vi "SIAM_to_ScanControl.vi"(8 "error in (no error)":errorcluster, 11 "Script":T3(array[cluster])=[{"Delay 10µs"=50, "command"=4060086273, "P0"=3, "P1"=2, "P2"=0, "P3"=0, "P4"=0, "P5-ticket"=0}, {"Delay 10µs"=0, "command"=101711937, "P0"=0, "P1"=627200, "P2"=0, "P3"=0, "P4"=0, "P5-ticket"=0}, {"Delay 10µs"=0, "command"=102760513, "P0"=0, "P1"=3851400, "P2"=0, "P3"=0, "P4"=0, "P5-ticket"=0}, {"Delay 10µs"=0, "command"=3289190402, "P0"=0, "P1"=0, "P2"=0, "P3"=0, "P4"=0, "P5-ticket"=0}, {"Delay 10µs"=264, "command"=102760481, "P0"=0, "P1"=0, "P2"=-1047728, "P3"=0, "P4"=0, "P5-ticket"=0}, {"Delay 10µs"=0, "command"=4060086273, "P0"=2, "P1"=7, "P2"=0, "P3"=0, "P4"=0, "P5-ticket"=0}, {"Delay 10µs"=116, "command"=3489660929, "P0"=2097152, "P1"=2097152, "P2"=0, "P3"=0, "P4"=0, "P5-ticket"=0}, {"Delay 10µs"=0, "command"=3489660929, "P0"=1, "P1"=1, "P2"=0, "P3"=0, "P4"=0, "P5-ticket"=0}, {"Delay 10µs"=100, "command"=3489660929, "P0"=1, "P1"=0, "P2"=0, "P3"=0, "P4"=0, "P5-ticket"=0}, {"Delay 10µs"=12638, "command"=3289190402, "P0"=0, "P1"=0, "P2"=0, "P3"=0, "P4"=0, "P5-ticket"=0}, {"Delay 10µs"=0, "command"=102760465, "P0"=0, "P1"=0, "P2"=0, "P3"=12718148, "P4"=0, "P5-ticket"=0}, {"Delay 10µs"=0, "command"=101711889, "P0"=0, "P1"=0, "P2"=0, "P3"=679161, "P4"=0, "P5-ticket"=0}, {"Delay 10µs"=132, "command"=102760465, "P0"=0, "P1"=0, "P2"=0, "P3"=-12718148, "P4"=0, "P5-ticket"=0}, {"Delay 10µs"=0, "command"=101711889, "P0"=0, "P1"=0, "P2"=0, "P3"=-679161, "P4"=0, "P5-ticket"=0}, {"Delay 10µs"=132, "command"=102760465, "P0"=0, "P1"=0, "P2"=0, "P3"=0, "P4"=0, "P5-ticket"=0}, {"Delay 10µs"=0, "command"=101711889, "P0"=0, "P1"=0, "P2"=0, "P3"=0, "P4"=0, "P5-ticket"=0}, {"Delay 10µs"=12855, "command"=3489660929, "P0"=2097152, "P1"=0, "P2"=0, "P3"=0, "P4"=0, "P5-ticket"=0}, {"Delay 10µs"=70, "command"=4043379297, "P0"=-7, "P1"=2, "P2"=1, "P3"=0, "P4"=0, "P5-ticket"=514}, {"Delay 10µs"=50, "command"=104857729, "P0"=-25600, "P1"=0, "P2"=0, "P3"=0, "P4"=0, "P5-ticket"=0}, {"Delay 10µs"=0, "command"=4043379297, "P0"=-43, "P1"=3, "P2"=1, "P3"=0, "P4"=0, "P5-ticket"=515}, {"Delay 10µs"=50, "command"=104857729, "P0"=51200, "P1"=0, "P2"=0, "P3"=0, "P4"=0, "P5-ticket"=0}, {"Delay 10µs"=50, "command"=102760513, "P0"=0, "P1"=3840000, "P2"=0, "P3"=0, "P4"=0, "P5-ticket"=0}, {"Delay 10µs"=10, "command"=4027518991, "P0"=0, "P1"=0, "P2"=0, "P3"=0, "P4"=0, "P5-ticket"=112}] {"command" format="%x" items=["read_x-Motor_status_ticket"=17305600, "init_x-Motor"=17760263, "read_x-Motor_absolute_ticket"=16781312, "move_x-Motor_absolute"=16777217, "move_x-Motor_relative"=16842753, "read_x-Motor_speed"=16977920, "set_x-Motor_speed"=16973825, "read_y-Motor_status_ticket"=18354176, "init_y-Motor"=18808839, "read_y-Motor_absolute_ticket"=17829888, "move_y-Motor_absolute"=17825793, "move_y-Motor_relative"=17891329, "read_y-Motor_speed"=18026496, "set_y-Motor_speed"=18022401, "read_z-Motor_status_ticket"=19402752, "init_z-Motor"=19857415, "stop_z-Motor"=19857423, "start_z-Motor"=19857422, "read_z-Motor_absolute_ticket"=18878464, "move_z-Motor_absolute"=18874369, "move_z-Motor_relative"=18939905, "read_Objective_status_ticket"=20451328, "init_Objective"=20905991, "read_Objective_absolute_ticket"=19927040, "move_Objective_absolute"=19922945, "move_Objective_relative"=19988481, "read_Objective-Motor_speed"=20123648, "set_Objective-Motor_speed"=20119553, "read_Filter_status_ticket"=21499904, "init_Filter"=21954567, "read_Filter_absolute_ticket"=20975616, "move_Filter_absolute"=20971521, "move_Filter_relative"=21037057, "read_Filter-Motor_speed"=21172224, "set_Filter-Motor_speed"=21168129, "read_Trans-Rad_status_ticket"=22548480, "init_Trans-Rad"=23003143, "read_Trans-Rad_absolute_ticket"=22024192, "move_Trans-Rad_absolute"=22020097, "move_Trans-Rad_relative"=22085633, "read_Trans-Motor_speed"=22220800, "set_Trans-Motor_speed"=22216705, "read_FRET_status_ticket"=23597056, "init_FRET"=24051719, "read_FRET_absolute_ticket"=23072768, "move_FRET_absolute"=23068673, "move_FRET_relative"=23134209, "read_FRET-Motor_speed"=23269376, "set_FRET-Motor_speed"=23265281, "read_SI-Rad_status_ticket"=24645632, "init_SI-Rad"=25100295, "read_SI-Rad_absolute_ticket"=24121344, "move_SI-Rad_absolute"=24117249, "move_SI-Rad_relative"=24182785, "read_SI-Rad_speed"=24317952, "set_SI-Rad_speed"=24313857, "I2C-write"=335544337, "I2C-read"=335548433, "UART0-VC-Baud-write"=469958673, "UART0-VC-Baud-read"=469962768, "UART0-VC-write"=469762065, "UART0-VC-write-Var"=469762067, "UART0-VC-read"=469766160, "UART0-VC-read-Var"=469766162, "UART1-TSM-Baud-read"=486739984, "UART1-TSM-write"=486539281, "UART1-TSM-write-ticket"=486543377, "UART1-TSM-write-var-binary"=486539283, "UART1-TSM-write-var-binary-ticket"=486543379, "UART1-TSM-read"=486543376, "UART1-TSM-read-var-binary"=486543378, "UART2-write"=503316497, "UART2-read"=503320592, "USB-UART0-write"=536870929, "USB-UART0-read"=536875024, "USB-UART0-Float-Bitschift"=537133073, "USB-UART0-read-Float"=536875234, "USB-UART0-write-Float"=536871139, "USB-UART0-read-Float"=536875250, "USB-UART0-write-Float"=536871155, "end_no_ticket"=4027514895, "end_ticket"=4027518991, "NoOp"=4060086272, "IO-read_bank0"=3489665024, "IO-write_bank0"=3489660929, "IO-read_bank1"=3506442240, "IO-write_bank1"=3506438145, "DA0-0_LED365"=2684354561, "DA0-1_LED385"=2685403137, "DA0-2_LED440"=2686451713, "DA0-3_LED470"=2687500289, "DA0-4_LED510"=2688548865, "DA0-5_LED550"=2689597441, "DA0-6_LED590"=2690646017, "DA0-7_LED640"=2691694593, "DA1-0_LED-R"=2701131777, "DA1-1_LED-G"=2702180353, "DA1-2_LED-B"=2703228929, "DA1-3_LED-AF"=2704277505, "DA1-4"=2705326081, "DA1-5"=2706374657, "DA1-6"=2707423233, "DA1-7"=2708471809, "DA2-Laser0"=2717908993, "DA2-Laser1"=2718957569, "DA2-Laser2"=2720006145, "DA2-Laser3"=2721054721, "DA2-Laser4"=2722103297, "Analog-read_AD0-0"=2818576384, "Analog-read-store_AD0-0"=2818572290, "IO-delay_bank0"=3489923073, "IO-delay_bank0_fromVar"=3489923075, "read_cam_clock"=3289124864, "store_cam_clock"=3289120770, "read_cam_phase"=3289190400, "store_cam_phase"=3289186306, "store_cam_phase-t"=3289190402, "Read ticks"=4026535936, "Read ticks to var"=4026535938, "Read IP"=4043313152, "Read IP into var"=4043313154, "Set IP from var"=4043309059, "Set IP from var, relative"=4043313155, "branchRel_if_equal"=4043374849, "decrement_branchRel_if_equal"=4043374945, "decrement_branchRel_if_greaterequal"=4043375201, "decrement_branchRel_if_greaterequal_withTicket"=4043379297, "decrement_branchRel_if_smaller"=4043375457, "increment_branchRel_if_smaller"=4043375473, "readVar"=4060090368, "writeVar"=4060086273, "copyVar0_from_var1"=4060086275, "math_addToVariable"=4076863488, "math_addVToVariable"=4076863489, "math_subToVariable"=4076863490, "math_subVToVariable"=4076863491, "math_multToVariable"=4076863492, "math_multvToVariable"=4076863493, "math_divideToVariable"=4076863494, "math_divideVToVariable"=4076863495, "math_modToVariable"=4076863496, "math_modVToVariable"=4076863497, "logic_and"=4093640704, "logic_or"=4093640706, "logic_xor"=4093640708, "bitshift"=4093640712, "set_1Galvo"=101712113, "set_x-Galvo"=102760689, "set_y-Galvo"=103809265, "set_z-Fokus"=104857841, "set_1Galvo_position-only"=101711937, "set_x-Galvo_position-only"=102760513, "set_y-Galvo_position-only"=103809089, "set_z-Fokus_position-only"=104857665, "set_x-Galvo_position-only_ticket"=102764609, "set_y-Galvo_position-only_ticket"=103813185, "set_z-Fokus_position-only_ticket"=104861761, "set_1Galvo_relativ-only"=101712001, "set_x-Galvo_relativ-only"=102760577, "set_y-Galvo_relativ-only"=103809153, "set_z-Fokus_relativ-only"=104857729, "set_1Galvo_speed-only"=101711905, "set_x-Galvo_speed-only"=102760481, "set_y-Galvo_speed-only"=103809057, "set_z-Fokus_speed-only"=104857633, "set_1Galvo_acc-only"=101711889, "set_x-Galvo_acc-only"=102760465, "set_y-Galvo_acc-only"=103809041, "set_z-Fokus_acc-only"=104857617, "read_1Galvo_ticket"=101716032, "read_x-Galvo_ticket"=102764608, "read_y-Galvo_ticket"=103813184, "read_z-Focus_ticket"=104861760, "x-Galvo_pos_fromVar"=102760515, "y-Galvo_pos_fromVar"=103809091, "z-Focus_pos_fromVar"=104857667, "Servo0"=67108865, "Servo0-enable"=68091911, "Servo0-disable"=68091919, "Servo1"=68157441, "Servo1-enable"=69140487, "Servo1-disable"=69140495, "Servo2-enable"=70189063, "Servo2"=69206017, "Servo3-enable"=71237639, "Servo3"=70254593, "x-ssi-init"=202309639, "x-ssi-disable"=202309647, "x-ssi-Bits"=201523201, "x-ssi-Read"=201330688, "x-ssi-ReadToVar"=201326594, "x-ssi-ReadToVar-ticket"=201330690, "y-ssi-init"=203358215, "y-ssi-disable"=203358223, "y-ssi-Bits"=202571777, "y-ssi-Read"=202379264, "y-ssi-ReadToVar"=202375170, "y-ssi-ReadToVat-ticket"=202379266]}) -> (0 "error out":errorcluster, 2 "Total 10µs ticks":u32=1000000, 3 "ScanSteuerung":T6(array[cluster])=[{"Time [10µs]"=0.0, "action"=enum."Abs", "channel"=enum."Digital", "value (/s)"=7.0}, {"Time [10µs]"=0.0, "action"=enum."LoopStart", "channel"=enum."Loop", "value (/s)"=10.0}, {"Time [10µs]"=50000.0, "action"=enum."Abs", "channel"=enum."Digital", "value (/s)"=1.0}, {"Time [10µs]"=100000.0, "action"=enum."Rel", "channel"=enum."GalvoX", "value (/s)"=2.0}, {"Time [10µs]"=100000.0, "action"=enum."LoopEnd", "channel"=enum."Loop", "value (/s)"=0.0}])   [LabVIEW 2011]
uses:
  ScanControl_Action.ctl
  ScanControl_Channel.ctl
  Drivers/SIAM/SIAM_command.ctl
panel:
  out "loopstarts":T1(array[cluster])
  in  "Hack, valid loopvars":u16[](array[numeric])=[2, 3]
  out "Last Command":i32
  # "OK working\ntodo \nloop var detect\ncorrect loop times  from jump points"
  # "relative timing"
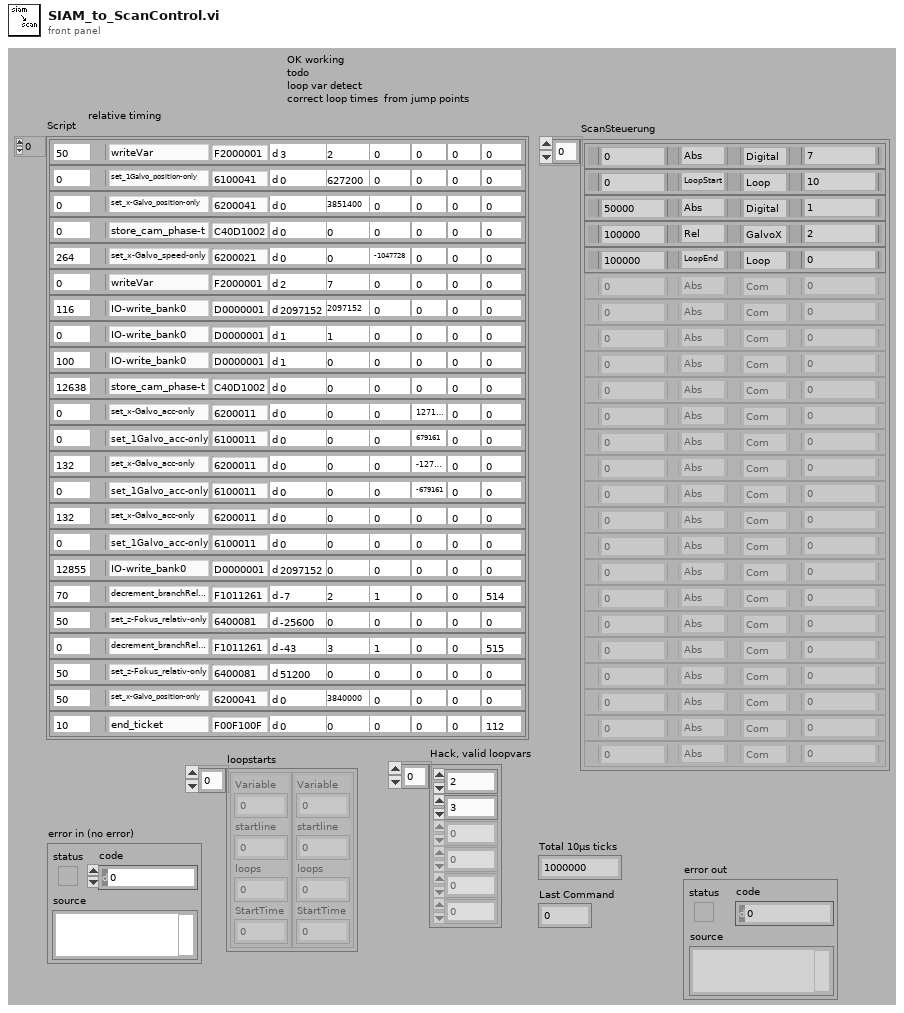
[diagram p1: front panel]
types:
  T1 = cluster{"Variable":i32, "startline":i32, "loops":i32, "StartTime":u64}[]
  T2 = typedef "SIAM_command.ctl" = u32
  T3 = cluster{"Delay 10µs":u32, "command":T2, "P0":i32, "P1":i32, "P2":i32, "P3":i32, "P4":i32, "P5-ticket":i32}[]
  T4 = typedef "ScanControl_Action.ctl" = enum16{"Abs", "Rel", "Inc", "IncInc", "LoopStart", "LoopEnd", "WaitTriggerRising"}
  T5 = typedef "ScanControl_Channel.ctl" = enum16{"Com", "AnalogConfig", "AnalogValue", "GalvoX", "GalvoY", "Galvo3", "Galvo4", "Digital", "Free", "Loop", "SMoveTime", "Image1X", "Image1Y", "Image2X", "Image2Y"}
  T6 = cluster{"Time [10µs]":dbl, "action":T4, "channel":T5, "value (/s)":dbl}[]
  T7 = cluster{"Time [10µs]":dbl, "action":T4, "channel":T5, "value (/s)":dbl}
  T8 = cluster{"Variable":i32, "startline":i32, "loops":i32, "StartTime":i32}[]
  T9 = enum16{"Com", "AnalogConfig", "AnalogValue", "GalvoX", "GalvoY", "Galvo3", "Galvo4", "Digital", "Free", "Loop", "SMoveTime", "Image1X", "Image1Y", "Image2X", "Image2Y"}[]
  T10 = enum8{"Ch0", "Ch1", "x-Galvo", "y-Galvo", "z-Focus"}
  T11 = cluster{"P0":i32, "startline":i32, "P1":i32, "StartTime":u64}[]
  T12 = cluster{"Variable":i32, "startline":i32, "loops":i32, "StartTime":u64}
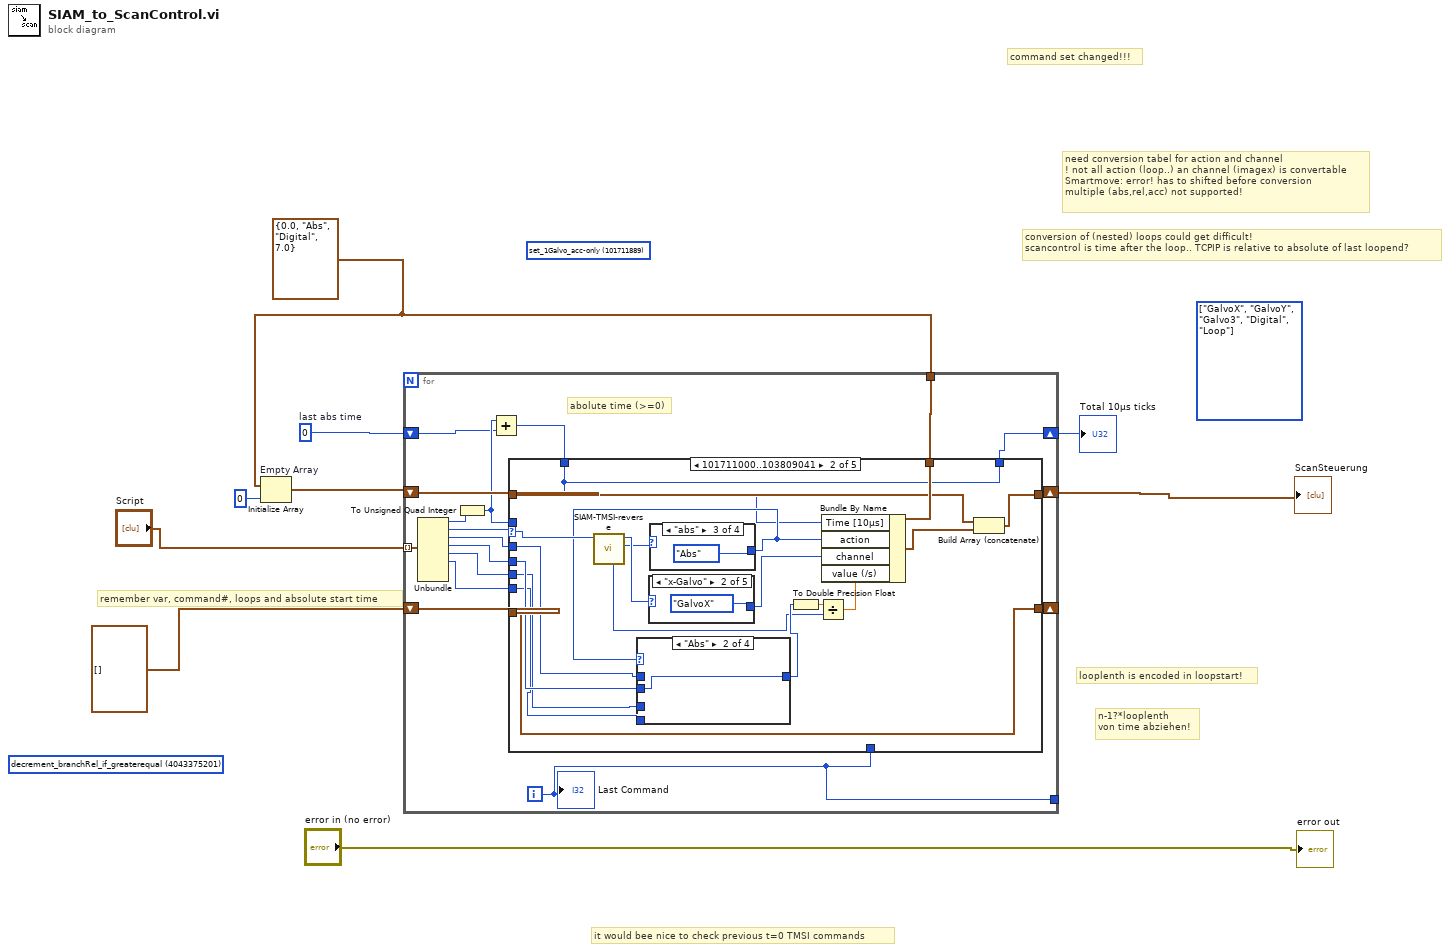
[diagram p0: block diagram]
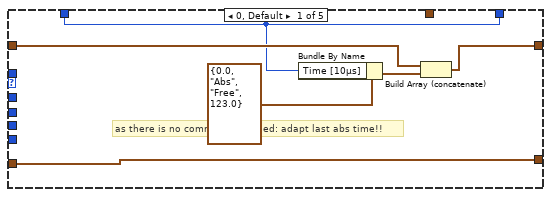
[diagram p2: hidden frame]
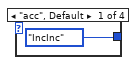
[diagram p6: hidden frame]
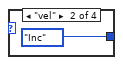
[diagram p7: hidden frame]
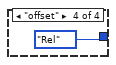
[diagram p8: hidden frame]
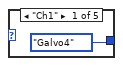
[diagram p9: hidden frame]
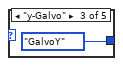
[diagram p10: hidden frame]
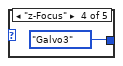
[diagram p11: hidden frame]
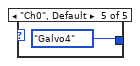
[diagram p12: hidden frame]
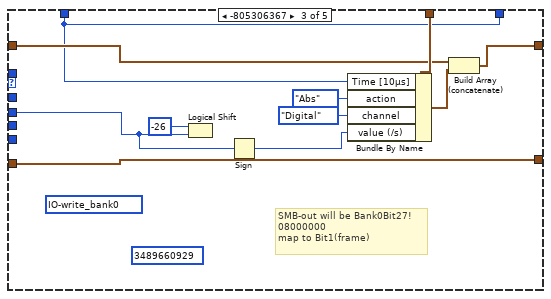
[diagram p13: hidden frame]
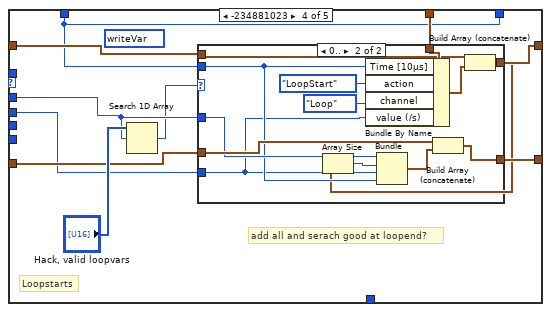
[diagram p14: hidden frame]
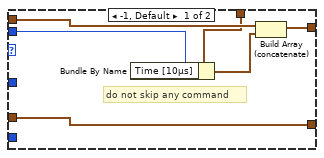
[diagram p15: hidden frame]
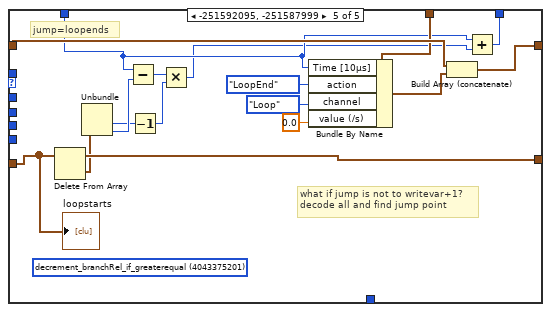
[diagram p16: hidden frame]
diagram:
  (unwired) T2 4043375201 items=["read_x-Motor_status_ticket"=17305600, "init_x-Motor"=17760263, "read_x-Motor_absolute_ticket"=16781312, "move_x-Motor_absolute"=16777217, "move_x-Motor_relative"=16842753, "read_y-Motor_status_ticket"=18354176, "init_y-Motor"=18808839, "read_y-Motor_absolute_ticket"=17829888, "move_y-Motor_absolute"=17825793, "move_y-Motor_relative"=17891329, "read_z-Motor_status_ticket"=19402752, "init_z-Motor"=19857415, "stop_z-Motor"=19857423, "start_z-Motor"=19857422, "read_z-Motor_absolute_ticket"=18878464, "move_z-Motor_absolute"=18874369, "move_z-Motor_relative"=18939905, "end_no_ticket"=4027514895, "end_ticket"=4027518991, "IO-read_bank0"=218107904, "IO-write_bank0"=218103809, "IO-read_bank1"=219156480, "IO-write_bank1"=219152385, "IO-delay_bank0"=218365953, "IO-delay_bank0_fromVar"=218365955, "read_cam_clock"=3289124864, "store_cam_clock"=3289120770, "read_cam_phase"=3289190400, "set_cam_deadtime"=3288989697, "set_cam_10uscycles"=3289055233, "set_cam_10uscycles_fromVariable"=3289055235, "calc_cam"=3289317386, "store_cam_Var"=3289251842, "math_addToVariable"=4060086278, "readVar"=4060090368, "writeVar"=4060086273, "copyVar"=4060086276, "decrement_branchRel_if_equal"=4043374945, "decrement_branchRel_if_greaterequal"=4043375201, "decrement_branchRel_if_greaterequal_withTicket"=4043379297, "decrement_branchRel_if_smaller"=4043375457, "increment_branchRel_if_smaller"=4043375473, "writeTMSI"=100663297, "writeTMSI_fromVar"=100663299] ("command")
  (unwired) T2 101711889 items=["read_x-Motor_status_ticket"=17305600, "init_x-Motor"=17760263, "read_x-Motor_absolute_ticket"=16781312, "move_x-Motor_absolute"=16777217, "move_x-Motor_relative"=16842753, "read_x-Motor_speed"=16977920, "set_x-Motor_speed"=16973825, "read_y-Motor_status_ticket"=18354176, "init_y-Motor"=18808839, "read_y-Motor_absolute_ticket"=17829888, "move_y-Motor_absolute"=17825793, "move_y-Motor_relative"=17891329, "read_y-Motor_speed"=18026496, "set_y-Motor_speed"=18022401, "read_z-Motor_status_ticket"=19402752, "init_z-Motor"=19857415, "stop_z-Motor"=19857423, "start_z-Motor"=19857422, "read_z-Motor_absolute_ticket"=18878464, "move_z-Motor_absolute"=18874369, "move_z-Motor_relative"=18939905, "read_Objective_status_ticket"=20451328, "init_Objective"=20905991, "read_Objective_absolute_ticket"=19927040, "move_Objective_absolute"=19922945, "move_Objective_relative"=19988481, "read_Objective-Motor_speed"=20123648, "set_Objective-Motor_speed"=20119553, "read_Filter_status_ticket"=21499904, "init_Filter"=21954567, "read_Filter_absolute_ticket"=20975616, "move_Filter_absolute"=20971521, "move_Filter_relative"=21037057, "read_Filter-Motor_speed"=21172224, "set_Filter-Motor_speed"=21168129, "read_Trans-Rad_status_ticket"=22548480, "init_Trans-Rad"=23003143, "read_Trans-Rad_absolute_ticket"=22024192, "move_Trans-Rad_absolute"=22020097, "move_Trans-Rad_relative"=22085633, "read_Trans-Motor_speed"=22220800, "set_Trans-Motor_speed"=22216705, "read_FRET_status_ticket"=23597056, "init_FRET"=24051719, "read_FRET_absolute_ticket"=23072768, "move_FRET_absolute"=23068673, "move_FRET_relative"=23134209, "read_FRET-Motor_speed"=23269376, "set_FRET-Motor_speed"=23265281, "read_SI-Rad_status_ticket"=24645632, "init_SI-Rad"=25100295, "read_SI-Rad_absolute_ticket"=24121344, "move_SI-Rad_absolute"=24117249, "move_SI-Rad_relative"=24182785, "read_SI-Rad_speed"=24317952, "set_SI-Rad_speed"=24313857, "I2C-write"=335544337, "I2C-read"=335548433, "UART0-VC-Baud-write"=469958673, "UART0-VC-Baud-read"=469962768, "UART0-VC-write"=469762065, "UART0-VC-write-Var"=469762067, "UART0-VC-read"=469766160, "UART0-VC-read-Var"=469766162, "UART1-TSM-Baud-read"=486739984, "UART1-TSM-write"=486539281, "UART1-TSM-write-ticket"=486543377, "UART1-TSM-write-var-binary"=486539283, "UART1-TSM-write-var-binary-ticket"=486543379, "UART1-TSM-read"=486543376, "UART1-TSM-read-var-binary"=486543378, "UART2-write"=503316497, "UART2-read"=503320592, "USB-UART0-write"=536870929, "USB-UART0-read"=536875024, "USB-UART0-Float-Bitschift"=537133073, "USB-UART0-read-Float"=536875234, "USB-UART0-write-Float"=536871139, "USB-UART0-read-Float"=536875250, "USB-UART0-write-Float"=536871155, "end_no_ticket"=4027514895, "end_ticket"=4027518991, "IO-read_bank0"=3489665024, "IO-write_bank0"=3489660929, "IO-read_bank1"=3506442240, "IO-write_bank1"=3506438145, "DA0-0_LED365"=2684354561, "DA0-1_LED385"=2685403137, "DA0-2_LED440"=2686451713, "DA0-3_LED470"=2687500289, "DA0-4_LED510"=2688548865, "DA0-5_LED550"=2689597441, "DA0-6_LED590"=2690646017, "DA0-7_LED640"=2691694593, "DA1-0_LED-R"=2701131777, "DA1-1_LED-G"=2702180353, "DA1-2_LED-B"=2703228929, "DA1-3_LED-AF"=2704277505, "DA1-4"=2705326081, "DA1-5"=2706374657, "DA1-6"=2707423233, "DA1-7"=2708471809, "DA2-Laser0"=2717908993, "DA2-Laser1"=2718957569, "DA2-Laser2"=2720006145, "DA2-Laser3"=2721054721, "DA2-Laser4"=2722103297, "Analog-read_AD0-0"=2818576384, "Analog-read-store_AD0-0"=2818572290, "IO-delay_bank0"=3489923073, "IO-delay_bank0_fromVar"=3489923075, "read_cam_clock"=3289124864, "store_cam_clock"=3289120770, "read_cam_phase"=3289190400, "store_cam_phase"=3289186306, "store_cam_phase-t"=3289190402, "Read ticks"=4027518976, "Read ticks to var"=4027518978, "Read IP"=4043313152, "Read IP into var"=4043313154, "Set IP from var"=4043309059, "Set IP from var, relative"=4043313155, "decrement_branchRel_if_equal"=4043374945, "decrement_branchRel_if_greaterequal"=4043375201, "decrement_branchRel_if_greaterequal_withTicket"=4043379297, "decrement_branchRel_if_smaller"=4043375457, "increment_branchRel_if_smaller"=4043375473, "readVar"=4060090368, "writeVar"=4060086273, "copyVar0_from_var1"=4060086275, "math_addToVariable"=4076863488, "math_addVToVariable"=4076863489, "math_subToVariable"=4076863490, "math_subVToVariable"=4076863491, "math_multToVariable"=4076863492, "math_multvToVariable"=4076863493, "math_divideToVariable"=4076863494, "math_divideVToVariable"=4076863495, "math_modToVariable"=4076863496, "math_modVToVariable"=4076863497, "logic_and"=4093640704, "logic_or"=4093640706, "logic_xor"=4093640708, "bitshift"=4093640712, "set_1Galvo"=101712113, "set_x-Galvo"=102760689, "set_y-Galvo"=103809265, "set_z-Fokus"=104857841, "set_1Galvo_position-only"=101711937, "set_x-Galvo_position-only"=102760513, "set_y-Galvo_position-only"=103809089, "set_z-Fokus_position-only"=104857665, "set_x-Galvo_position-only_ticket"=102764609, "set_y-Galvo_position-only_ticket"=103813185, "set_z-Fokus_position-only_ticket"=104861761, "set_1Galvo_relativ-only"=101712001, "set_x-Galvo_relativ-only"=102760577, "set_y-Galvo_relativ-only"=103809153, "set_z-Fokus_relativ-only"=104857729, "set_1Galvo_speed-only"=101711905, "set_x-Galvo_speed-only"=102760481, "set_y-Galvo_speed-only"=103809057, "set_z-Fokus_speed-only"=104857633, "set_1Galvo_acc-only"=101711889, "set_x-Galvo_acc-only"=102760465, "set_y-Galvo_acc-only"=103809041, "set_z-Fokus_acc-only"=104857617, "read_1Galvo_ticket"=101716032, "read_x-Galvo_ticket"=102764608, "read_y-Galvo_ticket"=103813184, "read_z-Focus_ticket"=104861760, "x-Galvo_pos_fromVar"=102760515, "y-Galvo_pos_fromVar"=103809091, "z-Focus_pos_fromVar"=104857667, "Servo0"=67108865, "Servo0-enable"=68091911, "Servo0-disable"=68091919, "Servo1"=68157441, "Servo1-enable"=69140487, "Servo1-disable"=69140495, "Servo2-enable"=70189063, "Servo2"=69206017, "Servo3-enable"=71237639, "Servo3"=70254593, "xEncoder-Enable"=202309639, "xEncoder-Bits"=201523201, "xEncoder-Read"=201330688, "xEncoder-Read"=201326594, "xEncoder-Read-ticket"=201330690, "yEncoder-Enable"=203358215, "yEncoder-Bits"=202571777, "yEncoder-Read"=202379264, "yEncoder-Read"=202375170, "yEncoder-Read-ticket"=202379266] ("command")
  w3 = T7 {"Time [10µs]"=0.0, "action"=enum."Abs", "channel"=enum."Digital", "value (/s)"=7.0} ("Cluster")
  (unwired) T9 [enum."GalvoX", enum."GalvoY", enum."Galvo3", enum."Digital", enum."Loop"] items=["Com", "AnalogConfig", "AnalogValue", "GalvoX", "GalvoY", "Galvo3", "Galvo4", "Digital", "Free", "Loop", "SMoveTime", "Image1X", "Image1Y", "Image2X", "Image2Y"] ("Aktiv")
  w9 = u64 0  # last abs time
  # "looplenth is encoded in loopstart!"
  # "it would bee nice to check previous t=0 TMSI commands"
  # "n-1?*looplenth\nvon time abziehen!"
  # "remember var, command#, loops and absolute start time"
  # "command set changed!!!"
  # "conversion of (nested) loops could get difficult!\nscancontrol is time after the loop.. TCPIP is relative to absolute of last loopend?"
  # "need conversion tabel for action and channel\n! not all action (loop..) an channel (imagex) is convertable\nSmartmove: error! has to shifted before conversion\nmultiple (abs,rel,acc) not supported!"
  n1 = Initialize Array "Empty Array"(w3, 0 ("dimension size")) -> (w8:T6)
  n2 = for {
    tunnel: "Script" -> [w18] mode=indexing
    shift-right: [w11] -> w6
    shift-left: w9 -> [w19]
    tunnel: w3 -> [w26]
    shift-right: [w24] -> w2
    shift-left: w8 -> [w25]
    shift-right: [w22] -> _
    shift-left: T8 [] -> [w23]
    tunnel: [w10] -> _
    i -> [w10]
    # "abolute time (>=0)"
    n3 = Unbundle(w18) -> ("Delay 10µs"=w21:u32, "command"=w17:T2, "P0"=w16:i32, "P1"=w15:i32, "P2"=w14:i32, "P3"=w12:i32)  [unwired: 2 out]
    n4 = To Unsigned Quad Integer(1:w21) -> (0:w20:u64)
    n5 = Add(x=w20, y=w19) -> (x+y=w13:u64)
    n6 = case shown="101711000..103809041" w17 {
      selector: w17 -> [_ w47 _ _ _]
      tunnel: w16 -> [_ w42 _ w81 _]
      tunnel: w15 -> [_ w41 w67 w76 _]
      tunnel: w14 -> [_ w40 _ _ _]
      tunnel: w26 -> [_ w51 w73 w85 w118]
      tunnel: w25 -> [w31 w50 w72 w84 w120]
      tunnel: [w30 w49 w75 w83 w119] -> w24
      tunnel: w13 -> [w27 w33 w65 w79 w107]
      tunnel: w23 -> [w32 w48 w71 w78 w108]
      tunnel: w20 -> [_ _ _ _ _]
      tunnel: [w32 w48 w71 w77 w114] -> w22
      tunnel: w12 -> [_ w38 _ _ _]
      tunnel: [w27 w33 w65 w79 w105] -> w11
      tunnel: w10 -> [_ _ _ _ _]
      frame 0, Default {
        # "as there is no command decoded: adapt last abs time!!"
        n7 = Bundle By Name(cluster=T7 {"Time [10µs]"=0.0, "action"=enum."Abs", "channel"=enum."Free", "value (/s)"=123.0} ("Cluster"), "Time [10µs]"=w27) -> (w28:T7)
        n8 = Build Array (concatenate)(w31, w28) -> (w30:T6)
      }
      frame 101711000..103809041 {
        n9 = call "SIAM-TMSI-reverse.vi"("command"=w47) -> ("Type"=w45:enum8{"acc", "vel", "abs", "offset"}, "Motor"=w46:T10, "Resolution-Factor"=w36:i32)  [unwired: 6 in, 2 out]
        n10 = case shown="\"x-Galvo\"" w46 {
          tunnel: [ScanControl_Channel."Galvo4" ("channel") ScanControl_Channel."GalvoX" ("channel") ScanControl_Channel."GalvoY" ("channel") ScanControl_Channel."Galvo3" ("channel") ScanControl_Channel."Galvo4" ("channel")] -> w43
          frame "Ch1" {
          }
          frame "x-Galvo" {
          }
          frame "y-Galvo" {
          }
          frame "z-Focus" {
          }
          frame "Ch0", Default {
          }
        }
        n11 = case shown="\"abs\"" w45 {
          tunnel: [ScanControl_Action."IncInc" ("action") ScanControl_Action."Inc" ("action") ScanControl_Action."Abs" ("action") ScanControl_Action."Rel" ("action")] -> w39
          frame "acc", Default {
          }
          frame "vel" {
          }
          frame "abs" {
          }
          frame "offset" {
          }
        }
        n12 = case shown="\"Abs\"" w39 {
          tunnel: w42 -> [w52 _ _ _]
          tunnel: w41 -> [_ w53 _ _]
          tunnel: w40 -> [_ _ w54 _]
          tunnel: w38 -> [_ _ _ w55]
          tunnel: [w52 w53 w54 w55] -> w37
          frame "Rel", Default {
          }
          frame "Abs" {
          }
          frame "Inc" {
          }
          frame "IncInc" {
          }
        }
        n13 = To Double Precision Float(number=w37) -> (double precision float=w34:dbl)
        n14 = Divide(x=w34, y=w36) -> (x/y=w35:dbl)
        n15 = Bundle By Name(cluster=w51, "Time [10µs]"=w33, "action"=w39, "channel"=w43, "value (/s)"=w35) -> (w44:T7)
        n16 = Build Array (concatenate)(w50, w44) -> (w49:T6)
      }
      frame -805306367 {
        (unwired) T2 3489660929 items=["read_x-Motor_status_ticket"=17305600, "init_x-Motor"=17760263, "read_x-Motor_absolute_ticket"=16781312, "move_x-Motor_absolute"=16777217, "move_x-Motor_relative"=16842753, "read_y-Motor_status_ticket"=18354176, "init_y-Motor"=18808839, "read_y-Motor_absolute_ticket"=17829888, "move_y-Motor_absolute"=17825793, "move_y-Motor_relative"=17891329, "read_z-Motor_status_ticket"=19402752, "init_z-Motor"=19857415, "stop_z-Motor"=19857423, "start_z-Motor"=19857422, "read_z-Motor_absolute_ticket"=18878464, "move_z-Motor_absolute"=18874369, "move_z-Motor_relative"=18939905, "end_no_ticket"=4027514895, "end_ticket"=4027518991, "IO-read_bank0"=3489665024, "IO-write_bank0"=3489660929, "IO-read_bank1"=3506442240, "IO-write_bank1"=3506438145, "IO-delay_bank0"=3489923073, "IO-delay_bank0_fromVar"=3489923075, "read_cam_clock"=3289124864, "store_cam_clock"=3289120770, "read_cam_phase"=3289190400, "set_cam_deadtime"=3288989697, "set_cam_10uscycles"=3289055233, "set_cam_10uscycles_fromVariable"=3289055235, "calc_cam"=3289317386, "store_cam_Var"=3289251842, "math_addToVariable"=4060086278, "readVar"=4060090368, "writeVar"=4060086273, "copyVar"=4060086276, "decrement_branchRel_if_equal"=4043374945, "decrement_branchRel_if_greaterequal"=4043375201, "decrement_branchRel_if_greaterequal_withTicket"=4043379297, "decrement_branchRel_if_smaller"=4043375457, "increment_branchRel_if_smaller"=4043375473, "set_x-Galvo"=1612710129, "set_y-Galvo"=1613758705, "set_z-Fokus"=1614807281, "set_x-Galvo_position-only"=1612709953, "set_y-Galvo_position-only"=1613758529, "set_z-Fokus_position-only"=1614807105, "set_x-Galvo_position-only_ticket"=1612714049, "set_y-Galvo_position-only_ticket"=1613762625, "set_z-Fokus_position-only_ticket"=1614811201, "read_x-Galvo_ticket"=1612714048, "read_y-Galvo_ticket"=1613762624, "read_z-Focus_ticket"=1614811200, "x-Galvo_pos_fromVar"=1612709955, "y-Galvo_pos_fromVar"=1613758531, "z-Focus_pos_fromVar"=1614807107] ("command")
        (unwired) u32 3489660929 ("data0")
        # "SMB-out will be Bank0Bit27!\n08000000\nmap to Bit1(frame)"
        n17 = Logical Shift(y=i8 -26, x=w67) -> ()  [unwired: 1 out]
        n18 = Sign(1:w67) -> (0:w66:i32)
        n19 = Bundle By Name(cluster=w73, "Time [10µs]"=w65, "action"=ScanControl_Action."Abs", "channel"=ScanControl_Channel."Digital", "value (/s)"=w66) -> (w74:T7)
        n20 = Build Array (concatenate)(w72, w74) -> (w75:T6)
      }
      frame -234881023 {
        (unwired) T2 4060086273 items=["read_x-Motor_status_ticket"=17305600, "init_x-Motor"=17760263, "read_x-Motor_absolute_ticket"=16781312, "move_x-Motor_absolute"=16777217, "move_x-Motor_relative"=16842753, "read_x-Motor_speed"=16977920, "set_x-Motor_speed"=16973825, "read_y-Motor_status_ticket"=18354176, "init_y-Motor"=18808839, "read_y-Motor_absolute_ticket"=17829888, "move_y-Motor_absolute"=17825793, "move_y-Motor_relative"=17891329, "read_y-Motor_speed"=18026496, "set_y-Motor_speed"=18022401, "read_z-Motor_status_ticket"=19402752, "init_z-Motor"=19857415, "stop_z-Motor"=19857423, "start_z-Motor"=19857422, "read_z-Motor_absolute_ticket"=18878464, "move_z-Motor_absolute"=18874369, "move_z-Motor_relative"=18939905, "read_Objective_status_ticket"=20451328, "init_Objective"=20905991, "read_Objective_absolute_ticket"=19927040, "move_Objective_absolute"=19922945, "move_Objective_relative"=19988481, "read_Objective-Motor_speed"=20123648, "set_Objective-Motor_speed"=20119553, "read_Filter_status_ticket"=21499904, "init_Filter"=21954567, "read_Filter_absolute_ticket"=20975616, "move_Filter_absolute"=20971521, "move_Filter_relative"=21037057, "read_Filter-Motor_speed"=21172224, "set_Filter-Motor_speed"=21168129, "read_Trans-Rad_status_ticket"=22548480, "init_Trans-Rad"=23003143, "read_Trans-Rad_absolute_ticket"=22024192, "move_Trans-Rad_absolute"=22020097, "move_Trans-Rad_relative"=22085633, "read_Trans-Motor_speed"=22220800, "set_Trans-Motor_speed"=22216705, "read_FRET_status_ticket"=23597056, "init_FRET"=24051719, "read_FRET_absolute_ticket"=23072768, "move_FRET_absolute"=23068673, "move_FRET_relative"=23134209, "read_FRET-Motor_speed"=23269376, "set_FRET-Motor_speed"=23265281, "read_SI-Rad_status_ticket"=24645632, "init_SI-Rad"=25100295, "read_SI-Rad_absolute_ticket"=24121344, "move_SI-Rad_absolute"=24117249, "move_SI-Rad_relative"=24182785, "read_SI-Rad_speed"=24317952, "set_SI-Rad_speed"=24313857, "I2C-write"=335544337, "I2C-read"=335548433, "UART0-VC-Baud-write"=469958673, "UART0-VC-Baud-read"=469962768, "UART0-VC-write"=469762065, "UART0-VC-write-Var"=469762067, "UART0-VC-read"=469766160, "UART0-VC-read-Var"=469766162, "UART1-TSM-Baud-read"=486739984, "UART1-TSM-write"=486539281, "UART1-TSM-write-ticket"=486543377, "UART1-TSM-write-var-binary"=486539283, "UART1-TSM-write-var-binary-ticket"=486543379, "UART1-TSM-read"=486543376, "UART1-TSM-read-var-binary"=486543378, "UART2-write"=503316497, "UART2-read"=503320592, "USB-UART0-write"=536870929, "USB-UART0-read"=536875024, "USB-UART0-Float-Bitschift"=537133073, "USB-UART0-read-Float"=536875234, "USB-UART0-write-Float"=536871139, "USB-UART0-read-Float"=536875250, "USB-UART0-write-Float"=536871155, "end_no_ticket"=4027514895, "end_ticket"=4027518991, "IO-read_bank0"=3489665024, "IO-write_bank0"=3489660929, "IO-read_bank1"=3506442240, "IO-write_bank1"=3506438145, "DA0-0_LED365"=2684354561, "DA0-1_LED385"=2685403137, "DA0-2_LED440"=2686451713, "DA0-3_LED470"=2687500289, "DA0-4_LED510"=2688548865, "DA0-5_LED550"=2689597441, "DA0-6_LED590"=2690646017, "DA0-7_LED640"=2691694593, "DA1-0_LED-R"=2701131777, "DA1-1_LED-G"=2702180353, "DA1-2_LED-B"=2703228929, "DA1-3_LED-AF"=2704277505, "DA1-4"=2705326081, "DA1-5"=2706374657, "DA1-6"=2707423233, "DA1-7"=2708471809, "DA2-Laser0"=2717908993, "DA2-Laser1"=2718957569, "DA2-Laser2"=2720006145, "DA2-Laser3"=2721054721, "DA2-Laser4"=2722103297, "Analog-read_AD0-0"=2818576384, "Analog-read-store_AD0-0"=2818572290, "IO-delay_bank0"=3489923073, "IO-delay_bank0_fromVar"=3489923075, "read_cam_clock"=3289124864, "store_cam_clock"=3289120770, "read_cam_phase"=3289190400, "store_cam_phase"=3289186306, "store_cam_phase-t"=3289190402, "Read ticks"=4027518976, "Read ticks to var"=4027518978, "Read IP"=4043313152, "Read IP into var"=4043313154, "Set IP from var"=4043309059, "Set IP from var, relative"=4043313155, "decrement_branchRel_if_equal"=4043374945, "decrement_branchRel_if_greaterequal"=4043375201, "decrement_branchRel_if_greaterequal_withTicket"=4043379297, "decrement_branchRel_if_smaller"=4043375457, "increment_branchRel_if_smaller"=4043375473, "readVar"=4060090368, "writeVar"=4060086273, "copyVar0_from_var1"=4060086275, "math_addToVariable"=4076863488, "math_addVToVariable"=4076863489, "math_subToVariable"=4076863490, "math_subVToVariable"=4076863491, "math_multToVariable"=4076863492, "math_multvToVariable"=4076863493, "math_divideToVariable"=4076863494, "math_divideVToVariable"=4076863495, "math_modToVariable"=4076863496, "math_modVToVariable"=4076863497, "logic_and"=4093640704, "logic_or"=4093640706, "logic_xor"=4093640708, "bitshift"=4093640712, "set_1Galvo"=101712113, "set_x-Galvo"=102760689, "set_y-Galvo"=103809265, "set_z-Fokus"=104857841, "set_1Galvo_position-only"=101711937, "set_x-Galvo_position-only"=102760513, "set_y-Galvo_position-only"=103809089, "set_z-Fokus_position-only"=104857665, "set_x-Galvo_position-only_ticket"=102764609, "set_y-Galvo_position-only_ticket"=103813185, "set_z-Fokus_position-only_ticket"=104861761, "set_1Galvo_relativ-only"=101712001, "set_x-Galvo_relativ-only"=102760577, "set_y-Galvo_relativ-only"=103809153, "set_z-Fokus_relativ-only"=104857729, "set_1Galvo_speed-only"=101711905, "set_x-Galvo_speed-only"=102760481, "set_y-Galvo_speed-only"=103809057, "set_z-Fokus_speed-only"=104857633, "set_1Galvo_acc-only"=101711889, "set_x-Galvo_acc-only"=102760465, "set_y-Galvo_acc-only"=103809041, "set_z-Fokus_acc-only"=104857617, "read_1Galvo_ticket"=101716032, "read_x-Galvo_ticket"=102764608, "read_y-Galvo_ticket"=103813184, "read_z-Focus_ticket"=104861760, "x-Galvo_pos_fromVar"=102760515, "y-Galvo_pos_fromVar"=103809091, "z-Focus_pos_fromVar"=104857667, "Servo0"=67108865, "Servo0-enable"=68091911, "Servo0-disable"=68091919, "Servo1"=68157441, "Servo1-enable"=69140487, "Servo1-disable"=69140495, "Servo2-enable"=70189063, "Servo2"=69206017, "Servo3-enable"=71237639, "Servo3"=70254593, "xEncoder-Enable"=202309639, "xEncoder-Bits"=201523201, "xEncoder-Read"=201330688, "xEncoder-Read"=201326594, "xEncoder-Read-ticket"=201330690, "yEncoder-Enable"=203358215, "yEncoder-Bits"=202571777, "yEncoder-Read"=202379264, "yEncoder-Read"=202375170, "yEncoder-Read-ticket"=202379266] ("command")
        # "add all and serach good at loopend?"
        # "Loopstarts"
        n21 = Search 1D Array(1D array="Hack, valid loopvars", element=w81) -> (index of element=w80:i32)  [unwired: 1 in]
        n22 = case shown="0.." w80 {
          tunnel: w79 -> [w87 w95]
          tunnel: w81 -> [_ w96]
          tunnel: w85 -> [w88 w102]
          tunnel: w84 -> [w91 w101]
          tunnel: [w89 w94] -> w83
          tunnel: w78 -> [w90 w99]
          tunnel: [w90 w98] -> w77
          tunnel: w76 -> [_ w92]
          frame -1, Default {
            # "do not skip any command"
            n23 = Bundle By Name(cluster=w88, "Time [10µs]"=w87) -> (w86:T7)
            n24 = Build Array (concatenate)(w91, w86) -> (w89:T6)
          }
          frame 0.. {
            n25 = Bundle By Name(cluster=w102, "Time [10µs]"=w95, "action"=ScanControl_Action."LoopStart", "channel"=ScanControl_Channel."Loop", "value (/s)"=w92) -> (w100:T7)
            n26 = Build Array (concatenate)(w101, w100) -> (w94:T6)
            n27 = Array Size(array=w94) -> (size(s)=w93:i32)
            n28 = Bundle("P0"=w96, w93, "P1"=w92, w95) -> (w97:cluster{"P0":i32, i32, "P1":i32, u64})  [unwired: 1 in]
            n29 = Build Array (concatenate)(w99, w97) -> (w98:T11)
          }
        }
      }
      frame -251592095, -251587999 {
        (unwired) T2 4043375201 items=["read_x-Motor_status_ticket"=17305600, "init_x-Motor"=17760263, "read_x-Motor_absolute_ticket"=16781312, "move_x-Motor_absolute"=16777217, "move_x-Motor_relative"=16842753, "read_x-Motor_speed"=16977920, "set_x-Motor_speed"=16973825, "read_y-Motor_status_ticket"=18354176, "init_y-Motor"=18808839, "read_y-Motor_absolute_ticket"=17829888, "move_y-Motor_absolute"=17825793, "move_y-Motor_relative"=17891329, "read_y-Motor_speed"=18026496, "set_y-Motor_speed"=18022401, "read_z-Motor_status_ticket"=19402752, "init_z-Motor"=19857415, "stop_z-Motor"=19857423, "start_z-Motor"=19857422, "read_z-Motor_absolute_ticket"=18878464, "move_z-Motor_absolute"=18874369, "move_z-Motor_relative"=18939905, "read_Objective_status_ticket"=20451328, "init_Objective"=20905991, "read_Objective_absolute_ticket"=19927040, "move_Objective_absolute"=19922945, "move_Objective_relative"=19988481, "read_Objective-Motor_speed"=20123648, "set_Objective-Motor_speed"=20119553, "read_Filter_status_ticket"=21499904, "init_Filter"=21954567, "read_Filter_absolute_ticket"=20975616, "move_Filter_absolute"=20971521, "move_Filter_relative"=21037057, "read_Filter-Motor_speed"=21172224, "set_Filter-Motor_speed"=21168129, "read_Trans-Rad_status_ticket"=22548480, "init_Trans-Rad"=23003143, "read_Trans-Rad_absolute_ticket"=22024192, "move_Trans-Rad_absolute"=22020097, "move_Trans-Rad_relative"=22085633, "read_Trans-Motor_speed"=22220800, "set_Trans-Motor_speed"=22216705, "read_FRET_status_ticket"=23597056, "init_FRET"=24051719, "read_FRET_absolute_ticket"=23072768, "move_FRET_absolute"=23068673, "move_FRET_relative"=23134209, "read_FRET-Motor_speed"=23269376, "set_FRET-Motor_speed"=23265281, "read_SI-Rad_status_ticket"=24645632, "init_SI-Rad"=25100295, "read_SI-Rad_absolute_ticket"=24121344, "move_SI-Rad_absolute"=24117249, "move_SI-Rad_relative"=24182785, "read_SI-Rad_speed"=24317952, "set_SI-Rad_speed"=24313857, "I2C-write"=335544337, "I2C-read"=335548433, "UART0-VC-Baud-write"=469958673, "UART0-VC-Baud-read"=469962768, "UART0-VC-write"=469762065, "UART0-VC-write-Var"=469762067, "UART0-VC-read"=469766160, "UART0-VC-read-Var"=469766162, "UART1-TSM-Baud-read"=486739984, "UART1-TSM-write"=486539281, "UART1-TSM-write-ticket"=486543377, "UART1-TSM-write-var-binary"=486539283, "UART1-TSM-write-var-binary-ticket"=486543379, "UART1-TSM-read"=486543376, "UART1-TSM-read-var-binary"=486543378, "UART2-write"=503316497, "UART2-read"=503320592, "USB-UART0-write"=536870929, "USB-UART0-read"=536875024, "USB-UART0-Float-Bitschift"=537133073, "USB-UART0-read-Float"=536875234, "USB-UART0-write-Float"=536871139, "USB-UART0-read-Float"=536875250, "USB-UART0-write-Float"=536871155, "end_no_ticket"=4027514895, "end_ticket"=4027518991, "IO-read_bank0"=3489665024, "IO-write_bank0"=3489660929, "IO-read_bank1"=3506442240, "IO-write_bank1"=3506438145, "DA0-0_LED365"=2684354561, "DA0-1_LED385"=2685403137, "DA0-2_LED440"=2686451713, "DA0-3_LED470"=2687500289, "DA0-4_LED510"=2688548865, "DA0-5_LED550"=2689597441, "DA0-6_LED590"=2690646017, "DA0-7_LED640"=2691694593, "DA1-0_LED-R"=2701131777, "DA1-1_LED-G"=2702180353, "DA1-2_LED-B"=2703228929, "DA1-3_LED-AF"=2704277505, "DA1-4"=2705326081, "DA1-5"=2706374657, "DA1-6"=2707423233, "DA1-7"=2708471809, "DA2-Laser0"=2717908993, "DA2-Laser1"=2718957569, "DA2-Laser2"=2720006145, "DA2-Laser3"=2721054721, "DA2-Laser4"=2722103297, "Analog-read_AD0-0"=2818576384, "Analog-read-store_AD0-0"=2818572290, "IO-delay_bank0"=3489923073, "IO-delay_bank0_fromVar"=3489923075, "read_cam_clock"=3289124864, "store_cam_clock"=3289120770, "read_cam_phase"=3289190400, "store_cam_phase"=3289186306, "store_cam_phase-t"=3289190402, "Read ticks"=4027518976, "Read ticks to var"=4027518978, "Read IP"=4043313152, "Read IP into var"=4043313154, "Set IP from var"=4043309059, "Set IP from var, relative"=4043313155, "decrement_branchRel_if_equal"=4043374945, "decrement_branchRel_if_greaterequal"=4043375201, "decrement_branchRel_if_greaterequal_withTicket"=4043379297, "decrement_branchRel_if_smaller"=4043375457, "increment_branchRel_if_smaller"=4043375473, "readVar"=4060090368, "writeVar"=4060086273, "copyVar0_from_var1"=4060086275, "math_addToVariable"=4076863488, "math_addVToVariable"=4076863489, "math_subToVariable"=4076863490, "math_subVToVariable"=4076863491, "math_multToVariable"=4076863492, "math_multvToVariable"=4076863493, "math_divideToVariable"=4076863494, "math_divideVToVariable"=4076863495, "math_modToVariable"=4076863496, "math_modVToVariable"=4076863497, "logic_and"=4093640704, "logic_or"=4093640706, "logic_xor"=4093640708, "bitshift"=4093640712, "set_1Galvo"=101712113, "set_x-Galvo"=102760689, "set_y-Galvo"=103809265, "set_z-Fokus"=104857841, "set_1Galvo_position-only"=101711937, "set_x-Galvo_position-only"=102760513, "set_y-Galvo_position-only"=103809089, "set_z-Fokus_position-only"=104857665, "set_x-Galvo_position-only_ticket"=102764609, "set_y-Galvo_position-only_ticket"=103813185, "set_z-Fokus_position-only_ticket"=104861761, "set_1Galvo_relativ-only"=101712001, "set_x-Galvo_relativ-only"=102760577, "set_y-Galvo_relativ-only"=103809153, "set_z-Fokus_relativ-only"=104857729, "set_1Galvo_speed-only"=101711905, "set_x-Galvo_speed-only"=102760481, "set_y-Galvo_speed-only"=103809057, "set_z-Fokus_speed-only"=104857633, "set_1Galvo_acc-only"=101711889, "set_x-Galvo_acc-only"=102760465, "set_y-Galvo_acc-only"=103809041, "set_z-Fokus_acc-only"=104857617, "read_1Galvo_ticket"=101716032, "read_x-Galvo_ticket"=102764608, "read_y-Galvo_ticket"=103813184, "read_z-Focus_ticket"=104861760, "x-Galvo_pos_fromVar"=102760515, "y-Galvo_pos_fromVar"=103809091, "z-Focus_pos_fromVar"=104857667, "Servo0"=67108865, "Servo0-enable"=68091911, "Servo0-disable"=68091919, "Servo1"=68157441, "Servo1-enable"=69140487, "Servo1-disable"=69140495, "Servo2-enable"=70189063, "Servo2"=69206017, "Servo3-enable"=71237639, "Servo3"=70254593, "xEncoder-Enable"=202309639, "xEncoder-Bits"=201523201, "xEncoder-Read"=201330688, "xEncoder-Read"=201326594, "xEncoder-Read-ticket"=201330690, "yEncoder-Enable"=203358215, "yEncoder-Bits"=202571777, "yEncoder-Read"=202379264, "yEncoder-Read"=202375170, "yEncoder-Read-ticket"=202379266] ("command")
        # "what if jump is not to writevar+1?\ndecode all and find jump point"
        # "jump=loopends"
        n30 = Delete From Array(array=w108) -> (deleted portion=w109:T12, array with subset deleted=w114:T1)  [unwired: 2 in]
        n31 = Unbundle(w109) -> ("loops"=w111:i32, "StartTime"=w113:u64)  [unwired: 2 out]
        n32 = Subtract(x=w107, y=w113) -> (x-y=w112:u64)
        n33 = Decrement(x=w111) -> (x-1=w110:i32)
        n34 = Multiply(x=w112, y=w110) -> (x*y=w106:u64)
        n35 = Bundle By Name(cluster=w118, "Time [10µs]"=w107, "action"=ScanControl_Action."LoopEnd", "channel"=ScanControl_Channel."Loop", "value (/s)"=0.0) -> (w121:T7)
        n36 = Build Array (concatenate)(w120, w121) -> (w119:T6)
        n37 = Add(x=w107, y=w106) -> (x+y=w105:u64)
        "loopstarts" <- w108
      }
    }
    "Last Command" <- w10
  }
  "ScanSteuerung" <- w2
  "Total 10µs ticks" <- w6
  "error out" <- "error in (no error)"
